vi "HTTP Server Class.vi"() -> ()   [LabVIEW 2020]
uses:
  HTTP Server/Server/Server.lvclass
panel:
  in  "HTTP Server":refnum<class "Server.lvclass">
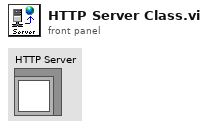
[diagram p1: front panel]
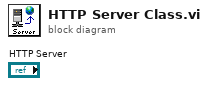
[diagram p0: block diagram]
diagram:
